vi "PM5000_VIF_Power_HMI.vi"(8 "error in":errorcluster, 11 "Network Path":string="172.22.26.202") -> (0 "error out":errorcluster, 2 "Generador1":T1 {"I1" scale=0.0..1200.0; "L1" scale=0.0..600.0; "Factor de Potencia" format="%#.1f"; "Potencia Total [kW]" format="%#.1f"; "Frecuencia [Hz]" format="%#.1f"; "I3" scale=0.0..1200.0; "I2" scale=0.0..1200.0; "L3" scale=0.0..600.0; "L2" scale=0.0..600.0}, 3 "Network Path out":string="192.168.169.1")   [LabVIEW 2018]
doc: "Lee la tabla de memoria RealTime_VIF_Power del equipo PowerMonitor 5000, ademas filtra y ordena las variables de interez de la tabla de memoria.\n\nLee las siguientes variables de la tabla RealTime_VIF_Power:\n\n*V1_V2_Volts\n*V2_V3_Volts\n*V3_V1_Volts\n*I1_Amps\n*I2_Amps\n*I3_Amps\n*Frequency_Hz\n*Total_kW\n*Total_kVAR\n*Total_kVA\n*Total_True_PF\n*Total_Disp_PF"
uses:
  Controls/Cluster_HMI_VIFP - 2.ctl
  <vilib>/RAFA Solutions/Harmony UI Controls Kit/Numeric/Horizontal Progress Bar.ctl
  <vilib>/RAFA Solutions/Harmony UI Controls Kit/Numeric/Numeric Indicator.ctl
  <vilib>/ethernetip/ethernetip.llb/EthernetIP SLC500 Read Float.vi
  <vilib>/ethernetip/ethernetip.lvlib
  <vilib>/RAFA Solutions/Harmony UI Controls Kit/Flat UI Design.lvlib
panel:
  # "VOLTAJES [Vrms]"
  # "CORRIENTES [Arms]"
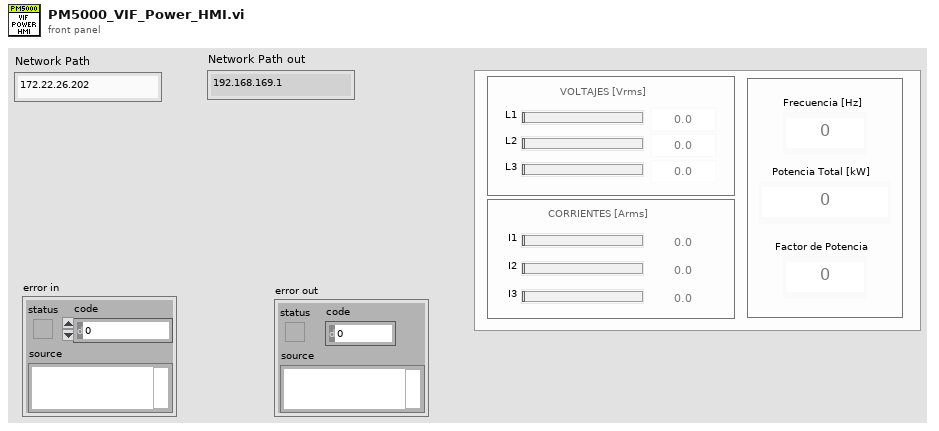
[diagram p1: front panel]
types:
  T1 = typedef "Cluster_HMI_VIFP - 2.ctl" = cluster{"L2":T2, "L3":T2, "I2":T2, "I3":T2, "Frecuencia [Hz]":T3, "Potencia Total [kW]":T3, "Factor de Potencia":T3, "L1":T2, "I1":T2}
  T2 = typedef "Flat UI Design.lvlib/Horizontal Progress Bar.ctl" = sgl
  T3 = typedef "Flat UI Design.lvlib/Numeric Indicator.ctl" = sgl
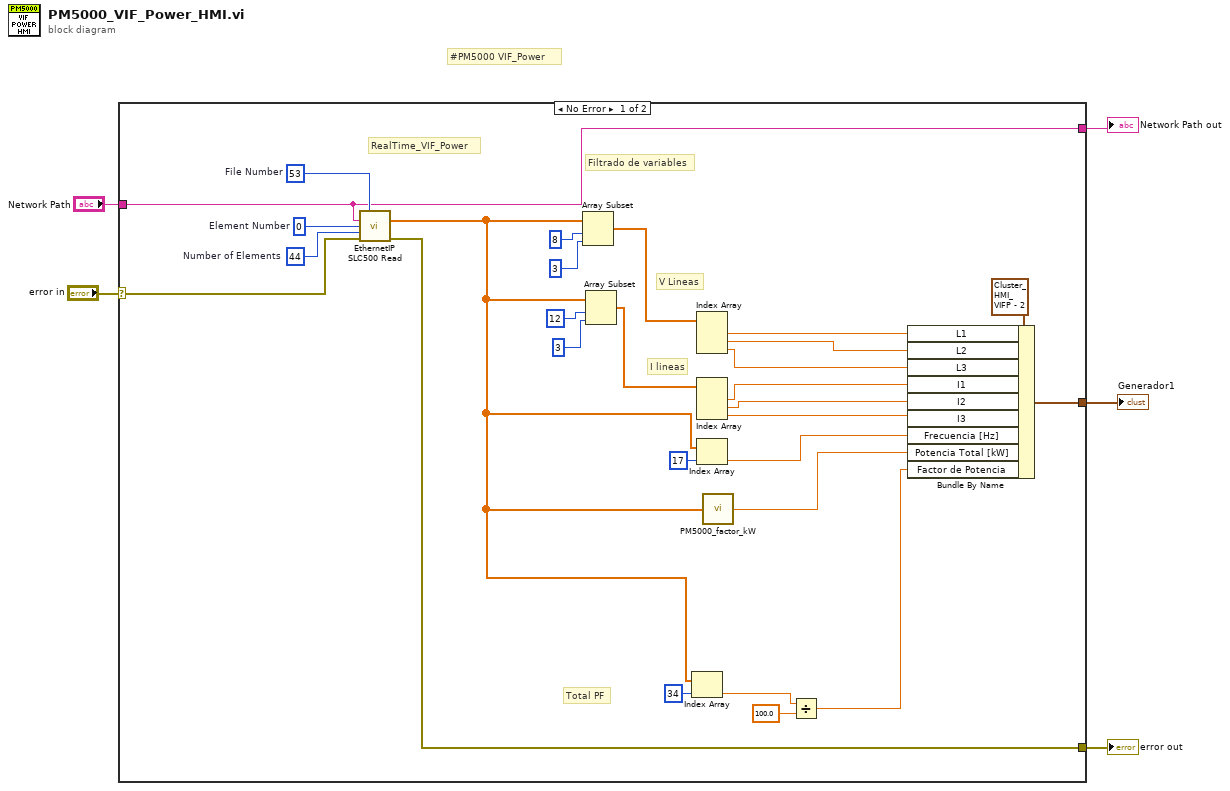
[diagram p0: block diagram]
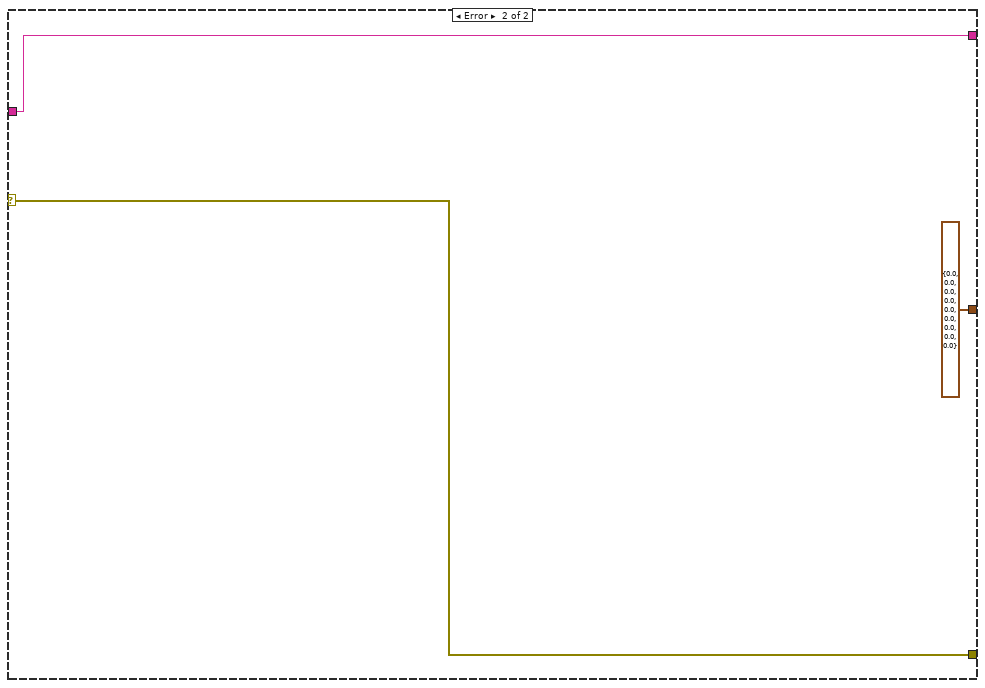
[diagram p2: hidden frame]
diagram:
  # "#PM5000 VIF_Power"
  n1 = case shown="No Error" "error in" {
    selector: "error in" -> [w25 w36]
    tunnel: [w30 w36] -> w5
    tunnel: [w22 w35] -> w3
    tunnel: "Network Path" -> [w22 w35]
    tunnel: [w11 T1 {"L2"=0.0, "L3"=0.0, "I2"=0.0, "I3"=0.0, "Frecuencia [Hz]"=0.0, "Potencia Total [kW]"=0.0, "Factor de Potencia"=0.0, "L1"=0.0, "I1"=0.0} ("Generador1")] -> w1
    frame No Error {
      w31 = u32 44  # Number of Elements
      w33 = u16 53  # File Number
      w32 = u16 0  # Element Number
      # "Total PF"
      # "I lineas"
      # "V Lineas"
      # "Filtrado de variables"
      # "RealTime_VIF_Power"
      n2 = call-poly <vilib>:"EthernetIP SLC500 Read.vi"("File Number"=w33, "Network Path"=w22, "Element Number"=w32, "Number of Elements"=w31, "error in"=w25) -> ("Data"=w7:sgl[], "error out"=w30:errorcluster)  [unwired: 8 in, 1 out]
      n3 = Array Subset(array=w7, index=8, length=3) -> (w24:sgl[])
      n4 = Array Subset(array=w7, index=12, length=3) -> (w23:sgl[])
      n5 = Index Array(array=w7, index=34) -> (element=w10:sgl)
      n6 = Index Array(array=w24) -> (element #1=w18:sgl, element #2=w17:sgl, element #3=w16:sgl)  [unwired: 3 in]
      n7 = Index Array(array=w23) -> (element #1=w15:sgl, element #2=w14:sgl, element #3=w13:sgl)  [unwired: 3 in]
      n8 = Index Array(array=w7, index=17) -> (element=w12:sgl)
      n9 = call "PM5000_factor_kW.vi"("Data In"=w7) -> ("kW"=w6:sgl)
      n10 = Divide(x=w10, y=sgl 100.0) -> (x/y=w8:sgl)
      n11 = Bundle By Name(cluster=T1 {"L2"=0.0, "L3"=0.0, "I2"=0.0, "I3"=0.0, "Frecuencia [Hz]"=0.0, "Potencia Total [kW]"=0.0, "Factor de Potencia"=0.0, "L1"=0.0, "I1"=0.0} ("Generador1"), "L1"=w18, "L2"=w17, "L3"=w16, "I1"=w15, "I2"=w14, "I3"=w13, "Frecuencia [Hz]"=w12, "Potencia Total [kW]"=w6, "Factor de Potencia"=w8) -> (w11:T1)
    }
    frame Error {
    }
  }
  "error out" <- w5
  "Network Path out" <- w3
  "Generador1" <- w1
